vi "Close.vi"(8 "error in (no error)":errorcluster, 11 "Xbox Controller in":refnum<class "Xbox Controller.lvclass">) -> (0 "error out":errorcluster)   [LabVIEW 2024, in "Xbox Controller.lvclass"]
doc: "MIT Licence\nCopyright (c) 2024 David Grollier"
uses:
  Xbox Controller.lvclass
  Xbox Controller.lvclass/Xbox Controller.ctl
  <vilib>/Utility/inputDevices.llb/closeJoystick.vi
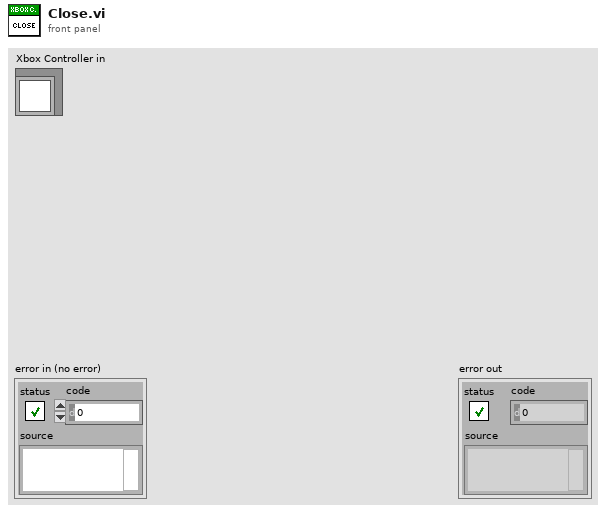
[diagram p1: front panel]
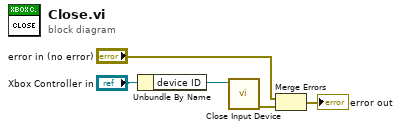
[diagram p0: block diagram]
diagram:
  n1 = Unbundle By Name("Xbox Controller in") -> ("device ID"=w4:refnum<k1>)
  n2 = call-poly <vilib>:"Close Input Device.vi"("device ID"=w4) -> ("error out"=w2:errorcluster)  [unwired: 9 in]
  n3 = Merge Errors("error in (no error)", w2) -> (→"error out":errorcluster)
